vi "ERIO RT Determine Server Update.vi"(8 "error in (no error)":errorcluster, 9 "Update Period (secs)":dbl=0.5, 11 "Supervisory Variables In":T1={"Alarm Threshold"=0.0, "Shutdown"=FALSE, "Enable SNS Alarm"=FALSE, "Enable SNS Stage Notification"=FALSE, "Enable SQS Notification"=FALSE, "Enable S3 TDMS Signal Capture"=FALSE, "Enable SystemLink Signal Capture"=FALSE, "Capture Signal"=FALSE, "Server Update"=FALSE, "AWS Access Key"="AKIAINLDO2Y2PDFEWDOQ", "AWS Secret Key"="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", "Phone Number"="+15037066913", "Region"=enum."us-west-2", "AWS SQS Queue"="mynicloud-demotest2", "AWS S3 Bucket"="mynicloud-demotest2"}) -> (0 "error out":errorcluster, 1 "Update Server":bool, 3 "Supervisory Variables Out":T1={"Alarm Threshold"=0.0, "Shutdown"=FALSE, "Enable SNS Alarm"=FALSE, "Enable SNS Stage Notification"=FALSE, "Enable SQS Notification"=FALSE, "Enable S3 TDMS Signal Capture"=FALSE, "Enable SystemLink Signal Capture"=FALSE, "Capture Signal"=FALSE, "Server Update"=FALSE, "AWS Access Key"="AKIAINLDO2Y2PDFEWDOQ", "AWS Secret Key"="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", "Phone Number"="+15037066913", "Region"=enum."us-west-2", "AWS SQS Queue"="mynicloud-demotest2", "AWS S3 Bucket"="mynicloud-demotest2"})   [LabVIEW 2017]
doc: "Check to see if it is time to update tags on the SystemLink server. \n\nJames Tillett P.E.\nEndeavor Engineering Inc.\nwww.endeavoreng.com"
uses:
  Controls/ERIO Supervisory Variables.ctl
  <vilib>/AWS Toolkit/Core/HTTP Request/Region.ctl
  <vilib>/AWS Toolkit/Core/HTTP Request/HTTP Request.lvclass
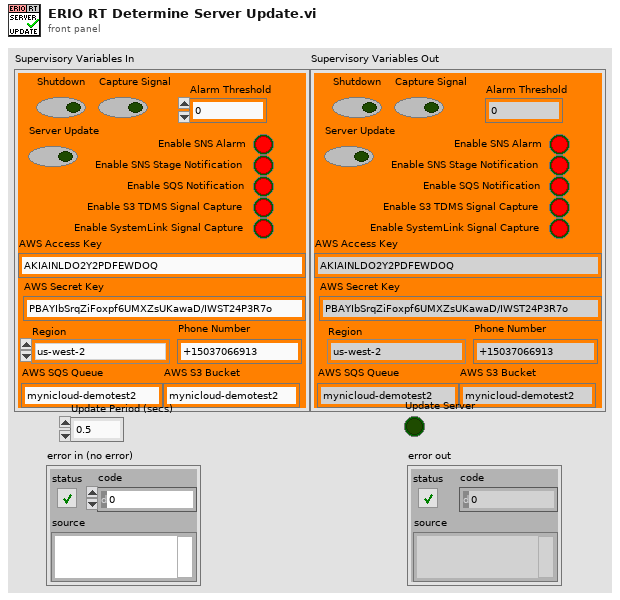
[diagram p1: front panel]
types:
  T1 = typedef "ERIO Supervisory Variables.ctl" = cluster{"Alarm Threshold":dbl, "Shutdown":bool, "Enable SNS Alarm":bool, "Enable SNS Stage Notification":bool, "Enable SQS Notification":bool, "Enable S3 TDMS Signal Capture":bool, "Enable SystemLink Signal Capture":bool, "Capture Signal":bool, "Server Update":bool, "AWS Access Key":string, "AWS Secret Key":string, "Phone Number":string, "Region":T2, "AWS SQS Queue":string, "AWS S3 Bucket":string}
  T2 = typedef "NI_AWS_Core.lvlib/HTTP Request.lvclass/Region.ctl" = enum16{"us-east-1", "us-east-2", "us-west-1", "us-west-2", "ap-northeast-1", "ap-northeast-2", "ap-southeast-1", "ap-southeast-2", "ca-central-1", "eu-central-1", "eu-west-1", "eu-west-2", "sa-east-1"}
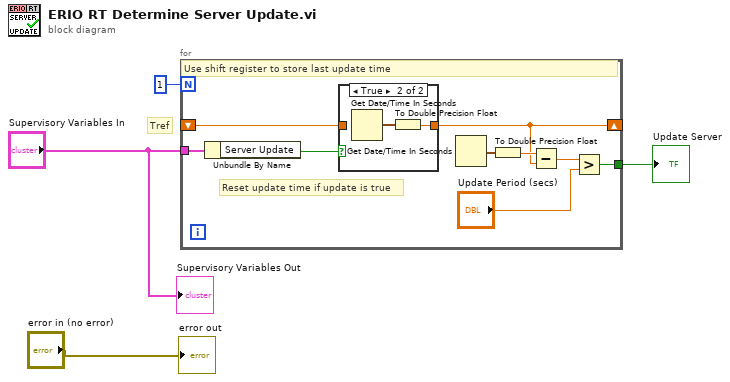
[diagram p0: block diagram]
diagram:
  # "Tref"
  n1 = for {
    N: 1 -> [_]
    shift-right: [w9] -> _
    shift-left: _ -> [w12]
    tunnel: "Supervisory Variables In" -> [w6]
    tunnel: [w5] -> w3
    # "Reset update time if update is true"
    # "Use shift register to store last update time"
    n2 = Unbundle By Name(w6) -> ("Server Update"=w13:bool)
    n3 = case shown="True" w13 {
      tunnel: [w14 w16] -> w9
      tunnel: w12 -> [w14 _]
      frame False {
      }
      frame True {
        n4 = Get Date/Time In Seconds() -> (seconds since 1Jan1904=w15:timestamp)
        n5 = To Double Precision Float(number=w15) -> (double precision float=w16:dbl)
      }
    }
    n6 = Get Date/Time In Seconds() -> (seconds since 1Jan1904=w11:timestamp)
    n7 = To Double Precision Float(number=w11) -> (double precision float=w10:dbl)
    n8 = Subtract(x=w10, y=w9) -> (x-y=w8:dbl)
    n9 = Greater?(x=w8, y="Update Period (secs)") -> (0:w5:bool)
  }
  "Update Server" <- w3
  "error out" <- "error in (no error)"
  "Supervisory Variables Out" <- "Supervisory Variables In"
